vi "Is a Search Prefix.vi"(1 "Constructor String Parser":T1) -> (0 "Is a Search Prefix?":bool)   [LabVIEW 2020, in "Stream.lvlib" / "URLPattern.lvclass"]
uses:
  URLPattern.lvclass
  Constructor String Parser.ctl
  Token.ctl
  Token Type.ctl
  URL Pattern Init.ctl
  Parser State.ctl
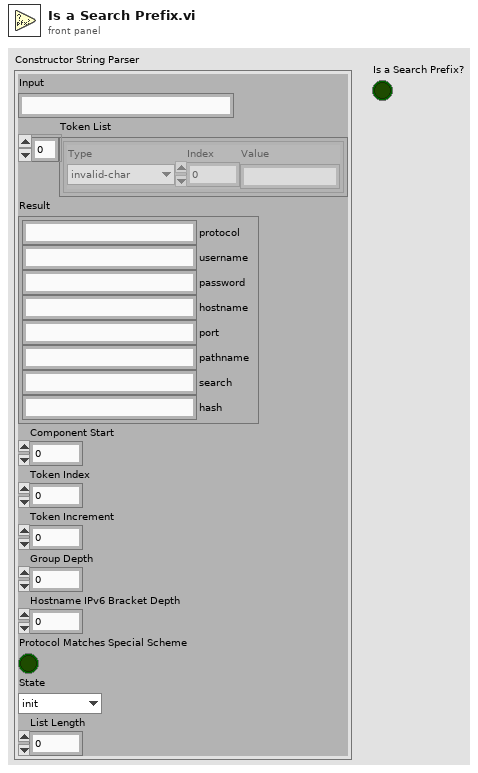
[diagram p1: front panel]
types:
  T1 = typedef "Stream.lvlib/URLPattern.lvclass/Constructor String Parser.ctl" = cluster{"Input":string, "Token List":T2[], "Result":T4, "Component Start":i32, "Token Index":i32, "Token Increment":i32, "Group Depth":i32, "Hostname IPv6 Bracket Depth":i32, "Protocol Matches Special Scheme":bool, "State":T5, "List Length":i32}
  T2 = typedef "Stream.lvlib/URLPattern.lvclass/Token.ctl" = cluster{"Type":T3, "Index":i32, "Value":string}
  T3 = typedef "Stream.lvlib/URLPattern.lvclass/Token Type.ctl" = enum16{"invalid-char", "open", "close", "regexp", "name", "char", "escaped-char", "other-modifier", "asterisk", "end"}
  T4 = typedef "Stream.lvlib/URLPattern.lvclass/URL Pattern Init.ctl" = cluster{"protocol":string, "username":string, "password":string, "hostname":string, "port":string, "pathname":string, "search":string, "hash":string}
  T5 = typedef "Stream.lvlib/URLPattern.lvclass/Parser State.ctl" = enum16{"init", "protocol", "authority", "username", "password", "hostname", "port", "pathname", "search", "hash", "done"}
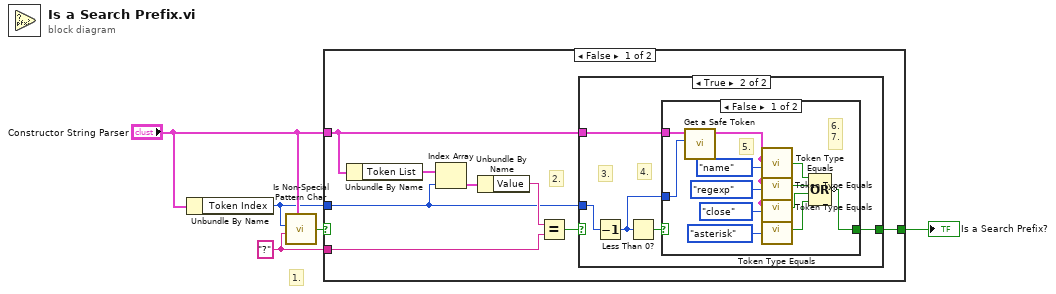
[diagram p0: block diagram]
diagram:
  w1 = "?" ("Value")
  # "1."
  n1 = Unbundle By Name("Constructor String Parser") -> ("Token Index"=w2:i32)
  n2 = call "Is Non-Special Pattern Char.vi"("Value"=w1, "Constructor String Parser"="Constructor String Parser", "Index"=w2) -> ("Non-Special Pattern Char?"=w4:bool)  [unwired: 7 in]
  n3 = case shown="False" w4 {
    selector: w4 -> [_ w33]
    tunnel: "Constructor String Parser" -> [w6 _]
    tunnel: [w8 w33] -> w3
    tunnel: w2 -> [w7 _]
    tunnel: w1 -> [w11 _]
    frame False {
      # "2."
      n4 = Unbundle By Name(w6) -> ("Token List"=w13:T2[])
      n5 = Index Array(array=w13, index=w7) -> (element=w12:T2)
      n6 = Unbundle By Name(w12) -> ("Value"=w10:string)
      n7 = Equal?(x=w10, y=w11) -> (x = y?=w9:bool)
      n8 = case shown="True" w9 {
        selector: w9 -> [w14 _]
        tunnel: [w14 w17] -> w8
        tunnel: w7 -> [_ w19]
        tunnel: w6 -> [_ w16]
        frame False {
        }
        frame True {
          # "4."
          # "3."
          n9 = Decrement(x=w19) -> (x-1=w15:i32)
          n10 = Less Than 0?(x=w15) -> (x < 0?=w18:bool)
          n11 = case shown="False" w18 {
            selector: w18 -> [_ w32]
            tunnel: [w20 w32] -> w17
            tunnel: w16 -> [w31 _]
            tunnel: w15 -> [w30 _]
            frame False {
              # "6.\n7."
              # "5."
              n12 = call "Get a Safe Token.vi"("Index"=w30, "Constructor String Parser"=w31) -> ("Token"=w25:T2)  [unwired: 8 in, 1 out]
              n13 = call "Token Type Equals.vi"("Type"=Token_Type."name", "Token"=w25) -> ("Type Equals?"=w24:bool)  [unwired: 2 in]
              n14 = call "Token Type Equals.vi"("Type"=Token_Type."regexp", "Token"=w25) -> ("Type Equals?"=w23:bool)  [unwired: 2 in]
              n15 = call "Token Type Equals.vi"("Type"=Token_Type."close", "Token"=w25) -> ("Type Equals?"=w22:bool)  [unwired: 2 in]
              n16 = call "Token Type Equals.vi"("Type"=Token_Type."asterisk", "Token"=w25) -> ("Type Equals?"=w21:bool)  [unwired: 2 in]
              n17 = Compound Arithmetic op=OR(w24, w23, w22, w21) -> (invert w20:bool)
            }
            frame True {
            }
          }
        }
      }
    }
    frame True {
    }
  }
  "Is a Search Prefix?" <- w3
